vi "Load Map.vi"(8 "error in (no error)":errorcluster, 11 "Map Model in":refnum<class "Map Model.lvclass">) -> (0 "error out":errorcluster, 3 "Map Model out":refnum<class "Map Model.lvclass">)   [LabVIEW 2020, in "Map Model.lvlib" / "Map Model.lvclass"]
uses:
  Map Model.lvclass
  Map Model.lvclass/Map Model.ctl
panel:
  # "NOTICE -- YOU MUST LEAVE THIS NOTICE IN PLACE.\n\nCopyright (c) 2017, LIANG LIU Shawn.Liu.cn@gmail.com\nAll rights reserved.\n\nRedistribution and use in source and binary forms, with or without modification, are permitted provided that the following conditions are met:\n-Redistributions of source code must retain the above copyright notice, this list of conditions and the following disclaimer.\n-Redistributions in binary form must reproduce the above copyright notice, this list of conditions and the following disclaimer in the documentation and/or other materials provided with the distribution.\n-Neither the name of the eLp nor the names of its contributors may be used to endorse or promote products derived from this software without specific prior written permission.\n\nTHIS SOFTWARE IS PROVIDED BY THE COPYRIGHT HOLDERS AND CONTRIBUTORS \"AS IS\" AND ANY EXPRESS OR IMPLIED WARRANTIES, INCLUDING, BUT NOT LIMITED TO, THE IMPLIED WARRANTIES OF MERCHANTABILITY AND FITNESS FOR A PARTICULAR PURPOSE ARE DISCLAIMED. IN NO EVENT SHALL THE COPYRIGHT HOLDER OR CONTRIBUTORS BE LIABLE FOR ANY DIRECT, INDIRECT, INCIDENTAL, SPECIAL, EXEMPLARY, OR CONSEQUENTIAL DAMAGES (INCLUDING, BUT NOT LIMITED TO, PROCUREMENT OF SUBSTITUTE GOODS OR SERVICES; LOSS OF USE, DATA, OR PROFITS; OR BUSINESS INTERRUPTION) HOWEVER CAUSED AND ON ANY THEORY OF LIABILITY, WHETHER IN CONTRACT, STRICT LIABILITY, OR TORT (INCLUDING NEGLIGENCE OR OTHERWISE) ARISING IN ANY WAY OUT OF THE USE OF THIS SOFTWARE, EVEN IF ADVISED OF THE POSSIBILITY OF SUCH DAMAGE."
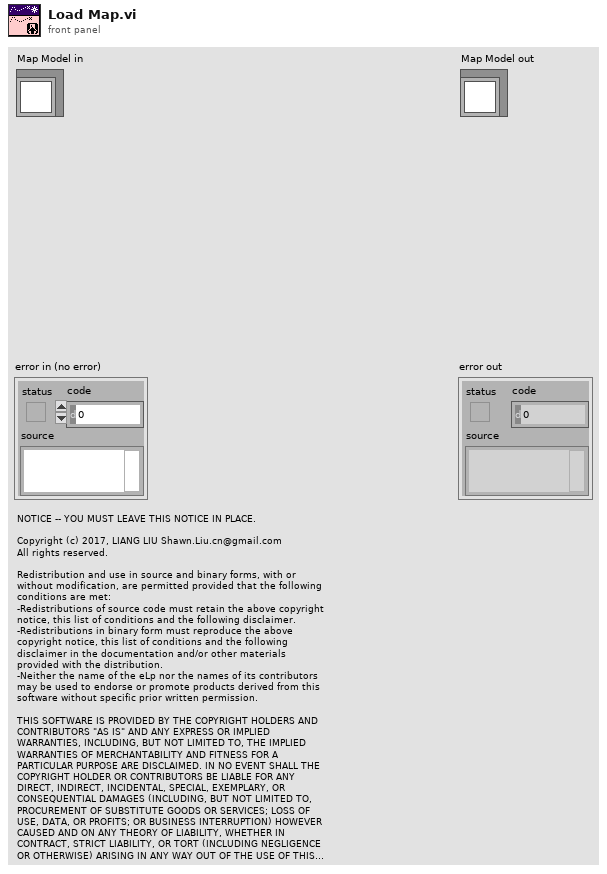
[diagram p1: front panel]
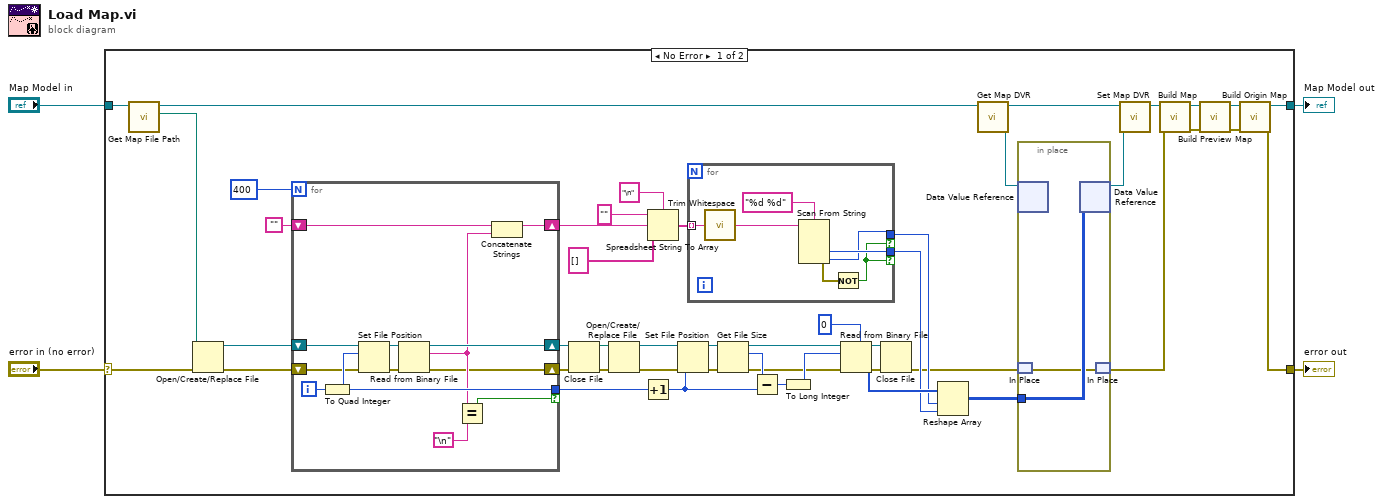
[diagram p0: block diagram]
diagram:
  n1 = case shown="No Error" "error in (no error)" {
    selector: "error in (no error)" -> [w50 w75]
    tunnel: "Map Model in" -> [w51 w74]
    tunnel: [w7 w74] -> w2
    tunnel: [w5 w75] -> w1
    frame No Error {
      n2 = call "Get Map File Path.vi"("Map Model in"=w51) -> ("Map File Path"=w10:path, "Map Model out"=w46:refnum<class "Map Model.lvclass">)  [unwired: 9 in]
      n3 = Open/Create/Replace File(file path (use dialog)=w10, error in=w50) -> (refnum out=w45:refnum<file>, error out=w20:errorcluster)  [unwired: 4 in, 1 out]
      n4 = for {
        N: 400 -> [_]
        shift-right: [w70] -> w42
        shift-left: w45 -> [w73]
        tunnel: [w68] -> w40 if=w67
        shift-right: [w65] -> w29
        shift-left: "" -> [w66]
        shift-right: [w61] -> w15
        shift-left: w20 -> [w63]
        i -> [w71]
        n5 = To Quad Integer(1:w71) -> (0:w68:i64)
        n6 = Set File Position(offset (in bytes) (0)=w68, refnum=w73, error in=w63) -> (refnum out=w72:refnum<file>, error out=w62:errorcluster)  [unwired: 1 in]
        n7 = Read from Binary File(8:w62, 11:w72) -> (0:w61:errorcluster, 2:w64:string, 3:w70:refnum<file>)  [unwired: 4 in, 1 out]
        n8 = Equal?(x=w64, y="\n") -> (x = y?=w67:bool)
        n9 = Concatenate Strings(w66, w64) -> (w65:string)
      }
      n10 = Close File(refnum=w42, error in=w15) -> (path=w41:path, error out=w19:errorcluster)
      n11 = Open/Create/Replace File(file path (use dialog)=w41, error in=w19) -> (refnum out=w39:refnum<file>, error out=w18:errorcluster)  [unwired: 4 in, 1 out]
      n12 = Increment(x=w40) -> (x+1=w35:i64)
      n13 = Spreadsheet String To Array(delimiter (Tab)="\n", format string="", spreadsheet string=w29, array type (2D Dbl)=string[] []) -> (array=w25:string[])
      n14 = Set File Position(offset (in bytes) (0)=w35, refnum=w39, error in=w18) -> (refnum out=w38:refnum<file>, error out=w17:errorcluster)  [unwired: 1 in]
      n15 = for {
        tunnel: w25 -> [w60] mode=indexing
        tunnel: [w57] -> w22 if=w55
        tunnel: [w56] -> w23 if=w55
        n16 = call <vilib>:"Trim Whitespace.vi"("string"=w60) -> ("trimmed string"=w59:string)  [unwired: 1 in]
        n17 = Scan From String(format string="%d %d", input string=w59) -> (error out=w54:errorcluster, output 1=w57:i32, output 2=w56:i32)  [unwired: 4 in, 2 out]
        n18 = Not(x=w54) -> (.not. x?=w55:bool)
      }
      n19 = Get File Size(file=w38, error in=w17) -> (refnum out=w37:refnum<file>, size (in bytes)=w36:i64, 0:w16:errorcluster)
      n20 = Subtract(x=w36, y=w35) -> (x-y=w34:i64)
      n21 = To Long Integer(number=w34) -> (32bit integer=w30:i32)
      n22 = Read from Binary File(5:u8 0, 8:w16, 10:w30, 11:w37) -> (0:w31:errorcluster, 2:w24:u8[], 3:w32:refnum<file>)  [unwired: 2 in, 1 out]
      n23 = Close File(refnum=w32, error in=w31) -> (error out=w12:errorcluster)  [unwired: 1 out]
      n24 = Reshape Array(w24, w23, w22) -> (w11:u8[][])
      n25 = call "Get Map DVR.vi"("Map Model in"=w46) -> ("Map DVR"=w13:refnum<data-value>, "Map Model out"=w21:refnum<class "Map Model.lvclass">)  [unwired: 9 in]
      n26 = in-place {
        in-place-border: w11 -> [w53]
        n27 = in-place-dvr #1(w13) -> ()  [unwired: 2 out]
        n28 = in-place-match #2(w12) -> (w52:errorcluster)
        n29 = in-place-dvr #1(w53) -> (w14:refnum<data-value>)  [unwired: 1 out]
        n30 = in-place-match #2(w52) -> (w9:errorcluster)
      }
      n31 = call "Set Map DVR.vi"("Map DVR"=w14, "Map Model in"=w21) -> ("Map Model out"=w47:refnum<class "Map Model.lvclass">)  [unwired: 9 in]
      n32 = call "Build Map.vi"("error in (no error)"=w9, "Map Model in"=w47) -> ("error out"=w8:errorcluster, "Map Model out"=w48:refnum<class "Map Model.lvclass">)  [unwired: 8 in]
      n33 = call "Build Preview Map.vi"("error in (no error)"=w8, "Map Model in"=w48) -> ("error out"=w6:errorcluster, "Map Model out"=w49:refnum<class "Map Model.lvclass">)  [unwired: 8 in]
      n34 = call "Build Origin Map.vi"("error in (no error)"=w6, "Map Model in"=w49) -> ("error out"=w5:errorcluster, "Map Model out"=w7:refnum<class "Map Model.lvclass">)  [unwired: 8 in]
    }
    frame Error {
    }
  }
  "error out" <- w1
  "Map Model out" <- w2
